vi "ToString.vi"(8 "error in (no error)":errorcluster, 11 "FakeTestCase in":refnum<class "FakeTestCase.lvclass">) -> (0 "error out":errorcluster, 2 "String":string, 3 "FakeTestCase out":refnum<class "FakeTestCase.lvclass">)   [LabVIEW 2017, in "ResultTreeListener.Tests.lvlib" / "Support.lvlib" / "FakeTestCase.lvclass"]
doc: "Returns the string representation for this object."
uses:
  FakeTestCase.lvclass
  FakeTestCase.lvclass/FakeTestCase.ctl
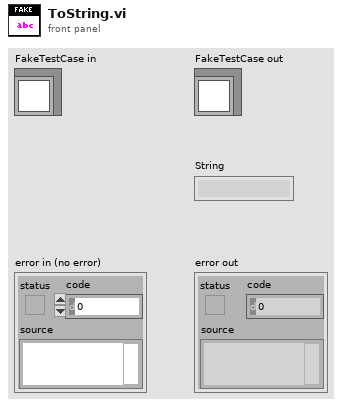
[diagram p1: front panel]
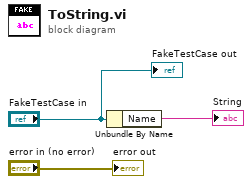
[diagram p0: block diagram]
diagram:
  n1 = Unbundle By Name("FakeTestCase in") -> ("Name"=→"String":string)
  "error out" <- "error in (no error)"
  "FakeTestCase out" <- "FakeTestCase in"
